vi "Cycle.vi"(11 "Start":T1[][](array[typedef])) -> (3 "Cycle array":T1[][](array[typedef]))   [LabVIEW 2023]
uses:
  ENUM_Type.ctl
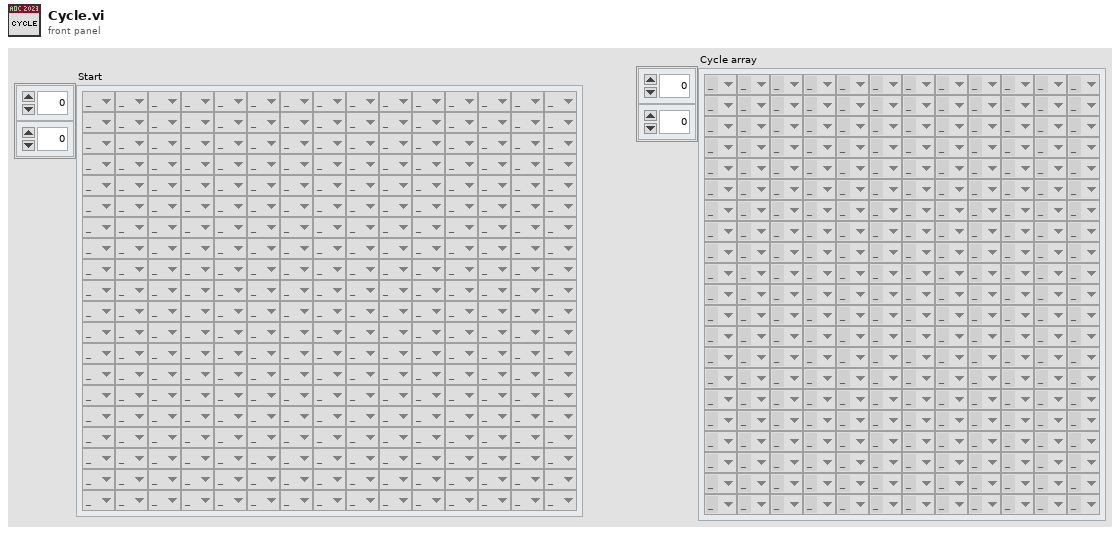
[diagram p1: front panel]
types:
  T1 = typedef "ENUM_Type.ctl" = enum16{"_", "O", "#"}
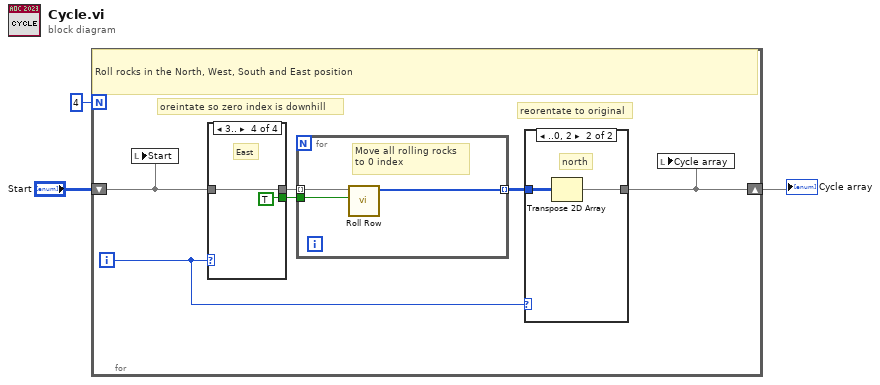
[diagram p0: block diagram]
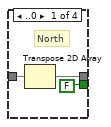
[diagram p3: hidden frame]
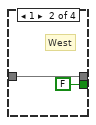
[diagram p4: hidden frame]
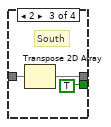
[diagram p5: hidden frame]
diagram:
  n1 = for {
    N: 4 -> [_]
    shift-right: [w4] -> w2
    shift-left: "Start" -> [w5]
    i -> [w6]
    # "reorentate to original"
    # "oreintate so zero index is downhill"
    # "Roll rocks in the North, West, South and East position"
    n2 = local write "Start"(w5) -> ()
    n3 = case shown="3.." w6 {
      tunnel: w5 -> [w15 w17 w20 w21]
      tunnel: [w14 w17 w19 w21] -> w9
      tunnel: [FALSE FALSE TRUE TRUE] -> w7
      frame ..0 {
        # "North"
        n4 = Transpose 2D Array(2D array=w15) -> (transposed array=w14:T1[][])
      }
      frame 1 {
        # "West"
      }
      frame 2 {
        # "South"
        n5 = Transpose 2D Array(2D array=w20) -> (transposed array=w19:T1[][])
      }
      frame 3.. {
        # "East"
      }
    }
    n6 = for {
      tunnel: w9 -> [w25] mode=indexing
      tunnel: [w24] -> w8 mode=indexing
      tunnel: w7 -> [w23]
      # "Move all rolling rocks\nto 0 index"
      n7 = call "Roll Row.vi"("Reverse"=w23, "Row In"=w25) -> ("Row Out"=w24:T1[])  [unwired: 9 in]
    }
    n8 = case shown="..0, 2" w6 {
      tunnel: w8 -> [w10 w12]
      tunnel: [w10 w11] -> w4
      frame 1, 3.. {
        # "West"
      }
      frame ..0, 2 {
        # "north"
        n9 = Transpose 2D Array(2D array=w12) -> (transposed array=w11:T1[][])
      }
    }
    n10 = local write "Cycle array"(w4) -> ()
  }
  "Cycle array" <- w2
